vi "basic_serial_write_and_read.vi"(0 "VISA resource name":refnum<visa-resource-name>="COM1", 1 "baud rate":u32=9600, 2 "data bits":u16=8 min=5 max=8 step=1, 3 "parity":u16(ring) items=["None", "Odd", "Even", "Mark", "Space"], 4 "stop bits":u16(ring)=10 items=["1.0"=10, "1.5"=15, "2.0"=20], 5 "write":bool=TRUE, 6 "read":bool=TRUE, 7 "flow control":u16(ring) items=["None"=0, "XON/XOFF"=1, "RTS/CTS"=2, "DTR/DSR"=4], 8 "string to write":string="*IDN?", 10 "bytes to read":u32=5) -> (9 "read string":string)   [LabVIEW 2013]
doc: "The Basic Serial Read and Write example performs a Serial Port Read, a Serial Port Write, or a combination of these actions. The user selects the actions (read or write) on the front panel. If both are selected, the VI will write the data first, read data, and then close the VISA session that is opened to the port. This VI will wait until the specified number of bytes is received at the port. Only the number of bytes specified will be read.\n\nINSTRUCTIONS:\n1) Select the serial resource and configuration parameters (baud rate, data bits, parity, stop bits, flow control).\n2) Select the operations to be performed. \n3) Connect the serial port to your device. If no device is available, perform a loopback test by doing one of the following. Short pins 2 and 3 on a RS-232 cable or short pin 4 to pin 8 and pin 5 to pin 9 on a RS-485/422 cable. \n4) Run the VI to see the data read. (The \"read string\" will match the \"string to write\" if a loopback test was performed.)\n\nNote: The parameters set for the serial port must match the parameters of the connected instrument or device. In this example, the bytes to read parameter specifies the number of bytes that the serial port reads. If there were more bytes at the port than the number specified in bytes to read, those bytes would not be read. Also, if you specify to read more bytes than the number of bytes actually read, you might receive a timeout error message.\n\nOn the block diagram, the Configure Serial Port VI sets the configuration parameters. The front panel displays the controls used to configure the basic parameters, such as baud rate, data bits, and parity. Constants configure the other parameters the user probably does not need set. After the VISA Configure Serial Port VI opens the VISA session and configures the port, the VI passes the VISA resource name to other VIs that perform operations on that VISA resource. The VISA Write function sends a command to the serial device and the VISA Read function returns data based on the command. The VISA Close function then closes the reference to the serial device. It is important to close the reference; otherwise communication through with that port through protocols other than VISA might not be possible."
uses:
  <vilib>/Instr/_visa.llb/VISA Configure Serial Port (Instr).vi
panel:
  # "Select the serial resource and the operations (Read, Write, or both) to be performed.  If both are selected, the VI will write the data first, read data and then close the VISA session that is opened to the port.  This VI will wait until the specified number of bytes is received at the port. Only the number of bytes specified will be read."
  # "For additional information select File >> VI Properties >> Documentation"
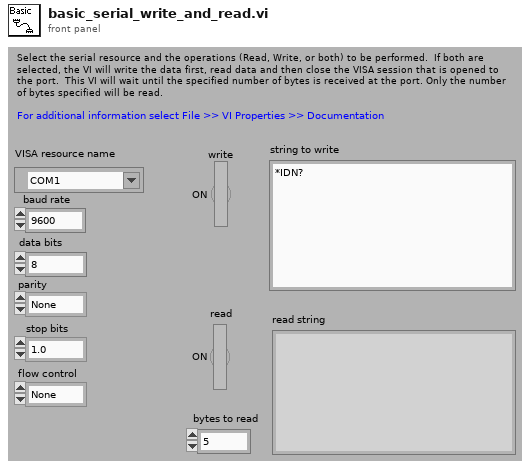
[diagram p1: front panel]
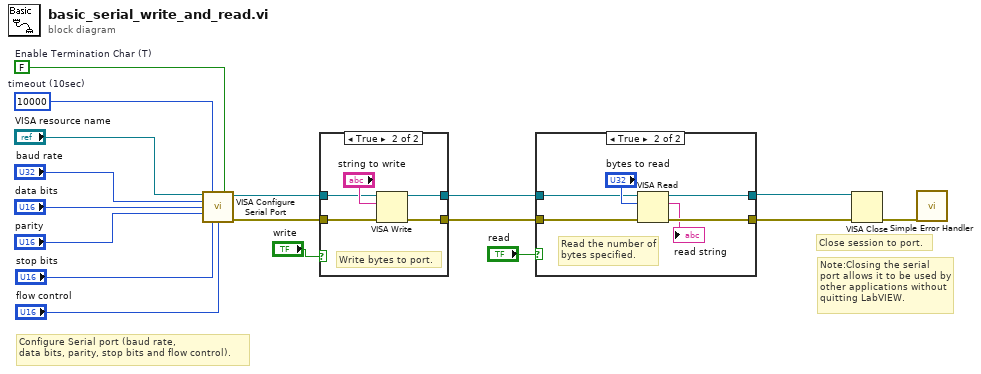
[diagram p0: block diagram]
diagram:
  w6 = FALSE  # Enable Termination Char (T)
  w7 = u32 10000  # timeout (10sec)
  # "Note:Closing the serial port allows it to be used by other applications without\nquitting LabVIEW."
  # "Configure Serial port (baud rate,\ndata bits, parity, stop bits and flow control)."
  # "Close session to port."
  n1 = call-poly "VISA Configure Serial Port"("VISA resource name"="VISA resource name", "timeout (10sec)"=w7, "Enable Termination\nChar (T)"=w6, "baud rate (9600)"="baud rate", "data bits (8)"="data bits", "parity (0:none)"="parity", "stop bits (10: 1 bit)"="stop bits", "flow control (0:none)"="flow control") -> ("VISA resource name out"=w13:refnum<visa-resource-name>, "error out"=w14:errorcluster)  [unwired: 6 in]
  n2 = case shown="True" "write" {
    tunnel: [w19 w24] -> w12
    tunnel: w13 -> [w18 w22]
    tunnel: w14 -> [w19 w21]
    tunnel: [w18 w20] -> w2
    frame False {
    }
    frame True {
      # "Write bytes to port."
      n3 = VISA Write(VISA resource name=w22, write buffer="string to write", error in (no error)=w21) -> (VISA resource name out=w20:refnum<visa-resource-name>, error out=w24:errorcluster)  [unwired: 1 out]
    }
  }
  n4 = case shown="True" "read" {
    tunnel: w12 -> [w26 w29]
    tunnel: [w26 w32] -> w11
    tunnel: [w25 w31] -> w10
    tunnel: w2 -> [w25 w27]
    frame False {
    }
    frame True {
      # "Read the number of bytes specified."
      n5 = VISA Read(VISA resource name=w27, byte count="bytes to read", error in (no error)=w29) -> (VISA resource name out=w31:refnum<visa-resource-name>, read buffer=→"read string":string, error out=w32:errorcluster)  [unwired: 1 out]
    }
  }
  n6 = VISA Close(VISA resource name=w10, error in (no error)=w11) -> (error out=w9:errorcluster)
  n7 = call <vilib>:"Simple Error Handler.vi"("error in (no error)"=w9) -> ()  [unwired: 4 in, 5 out]
